vi "replaceCategoryUpdateConditionToken.vi"(8 "error in (no error)":errorcluster, 10 "Query In":string, 11 "Transaction in":refnum<class "Transaction.lvclass">) -> (0 "error out":errorcluster, 2 "Query Out":string, 3 "Transaction out":refnum<class "Transaction.lvclass">)   [LabVIEW 2020]
uses:
  Transaction.lvclass
  Transaction.lvclass/Transaction.ctl
  C:/GitRepos/Filthy-Lucre-Budgetizer/source/support/classes/Transaction/Transaction.lvclass
  C:/GitRepos/Filthy-Lucre-Budgetizer/source/support/classes/RowDisplayable/RowRepresentable.lvclass
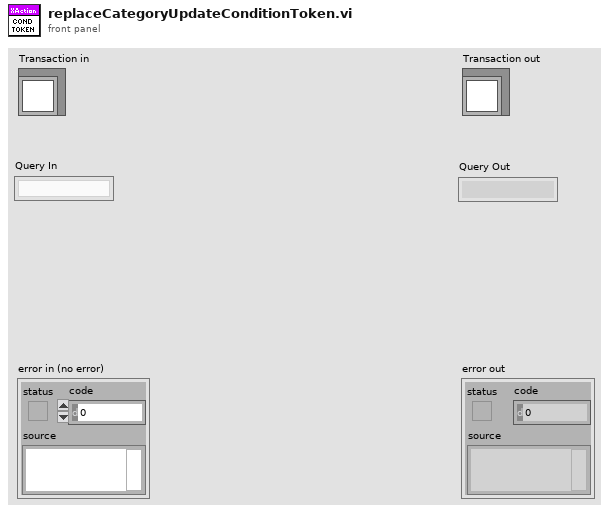
[diagram p1: front panel]
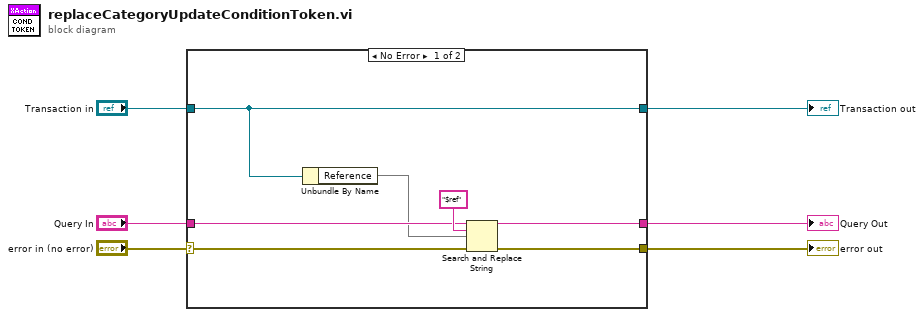
[diagram p0: block diagram]
diagram:
  n1 = case shown="No Error" "error in (no error)" {
    selector: "error in (no error)" -> [w12 w14]
    tunnel: [w11 w14] -> w5
    tunnel: [w9 w16] -> w3
    tunnel: "Transaction in" -> [w9 w16]
    tunnel: "Query In" -> [w10 w15]
    tunnel: [w7 w15] -> w1
    frame No Error {
      n2 = Unbundle By Name(w9) -> ("Reference"=w8)
      n3 = Search and Replace String(input string=w10, search string="$ref", replace string=w8, error in=w12) -> (result string=w7:string, error out=w11:errorcluster)  [unwired: 4 in, 2 out]
    }
    frame Error {
    }
  }
  "error out" <- w5
  "Transaction out" <- w3
  "Query Out" <- w1
